vi "QR  Code.vi"(0 "Session In":T1, 5 "Image In":T2, 11 "error in":errorcluster) -> (4 "Session Out":T1, 6 "Found?":bool, 8 "Image":T2(plugin-control), 10 "Data":string, 15 "error out":errorcluster)   [LabVIEW 2020]
doc: "Captures an Image and determines if QR Code is present. If QR Code is present in the image then the Data of the QR code is shown along with a boolean \"Found?\" to show if it was found or not. This can help when debugging."
uses:
  <vilib>/vision/Image Controls.llb/IMAQ Image.ctl
  <vilib>/userdefined/High Color/IMAQdx.ctl
  <vilib>/vision/NI_Vision_Development_Module.lvlib
  <vilib>/vision/driver/NI_Vision_Acquisition_Software.lvlib
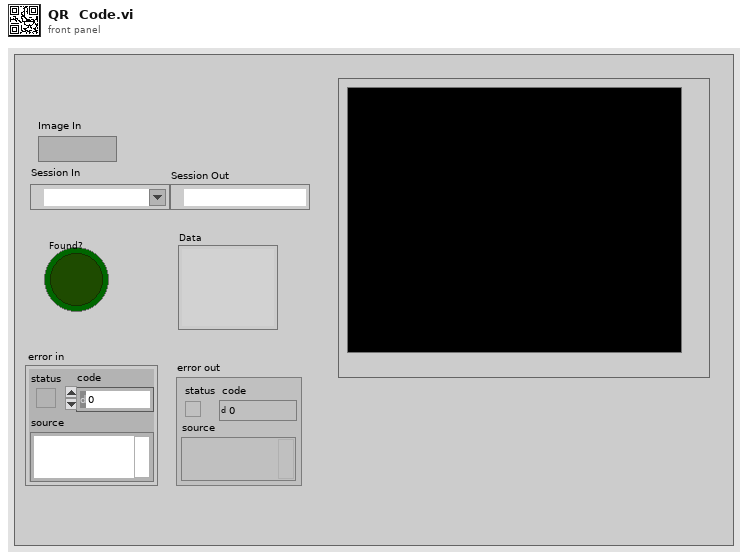
[diagram p1: front panel]
types:
  T1 = typedef "IMAQdx.ctl" = refnum<k21>
  T2 = typedef "IMAQ Image.ctl" = refnum<image>
  T3 = typedef "Image Type" = u32
  T4 = typedef "QR Code Report.ctl" = cluster{"Found?":bool, "Data":string, "Bounding Box":cluster{"x":sgl, "y":sgl}[], "Errors Corrected":u32, "Dimensions (Rows/Cols)":u32, "Version":u32, "QR Model":T5, "Stream Mode":T6, "Barcode Polarity":T7, "Mirrored?":bool, "Append Stream Position":u32, "Size of Append Stream":u32, "First EAN-128 ID":i32, "First Alternate Language ID":i32, "Append Stream ID":u32, "Minimum Edge Strength":u32, "Demodulation Mode":T8, "Cell Sample Size":T9, "Cell Filter Mode":T10}
  T5 = typedef "QR Code Model Type.ctl" = i32
  T6 = typedef "QR Code Stream Mode Type.ctl" = i32
  T7 = typedef "Data Matrix Polarity.ctl" = i32
  T8 = typedef "Demodulation Mode.ctl" = i32
  T9 = typedef "Cell Sample Size.ctl" = i32
  T10 = typedef "Cell Filter Mode.ctl" = i32
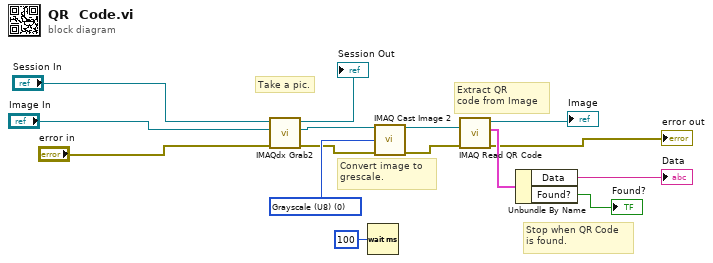
[diagram p0: block diagram]
diagram:
  w15 = T3 0 items=["Grayscale (U8)", "Grayscale (I16)", "Grayscale (SGL)", "Complex (CSG)", "RGB (U32)", "HSL (U32)", "RGB (U64)", "Grayscale (U16)"] ("Image Type")
  # "Stop when QR Code\nis found."
  # "Extract QR \ncode from Image"
  # "Convert image to \ngrescale."
  # "Take a pic."
  n1 = call <vilib>:"IMAQdx Grab2.vi"("error in"="error in", "Image In"="Image In", "Session In"="Session In") -> ("error out"=w11:errorcluster, "Image Out"=w10:T2, "Session Out"=→"Session Out":T1)  [unwired: 5 in, 1 out]
  n2 = Wait (ms)(milliseconds to wait=u32 100) -> ()  [unwired: 1 out]
  n3 = call "IMAQ Cast Image 2"("Image Src"=w10, "Image Type"=w15, "error in (no error)"=w11) -> ("Image Dst Out"=w9:T2, "error out"=w14:errorcluster)  [unwired: 11 in]
  n4 = call "IMAQ Read QR Code"("error in (no error)"=w14, "Image"=w9) -> ("error out"=→"error out":errorcluster, "QR Code Report"=w13:T4, "Image (duplicate)"=→"Image":T2)  [unwired: 6 in, 1 out]
  n5 = Unbundle By Name(w13) -> ("Data"=→"Data":string, "Found?"=→"Found?":bool)
